vi "Tool Q LEIN stroke Stop Pressure Monitoring.vi"(1 "Retry on err (F)":bool, 11 "error in (no error)":errorcluster) -> (4 "LEIN custom reply Q":T1, 15 "error out":errorcluster)   [LabVIEW 2011]
uses:
  LEINmaster/Defenitions/LEIN custom reply Q.ctl
  LEINmaster/Defenitions/LEIN Reply Holder.ctl
  LEINmaster/Defenitions/LEIN CMD Cluster.ctl
  LEINmaster/Defenitions/LEIN CMD List.ctl
  LEINmaster/Defenitions/LEIN Structure variations.ctl
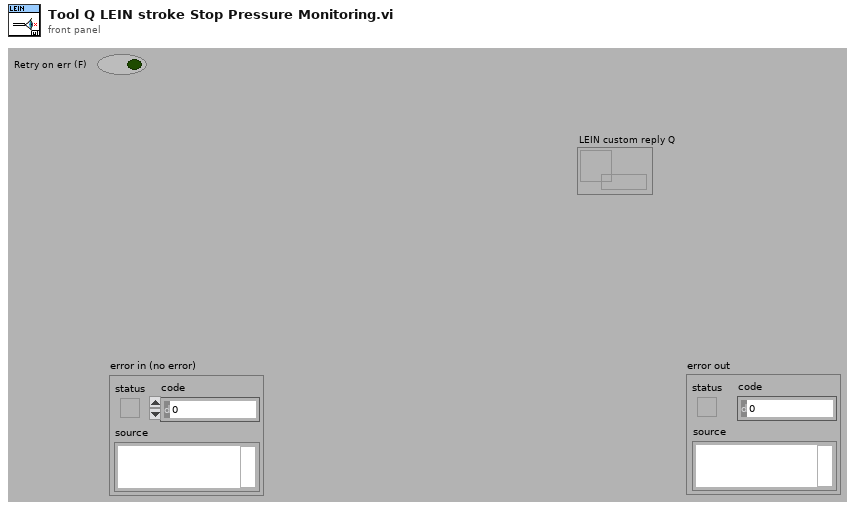
[diagram p1: front panel]
types:
  T1 = typedef "LEIN custom reply Q.ctl" = refnum<queue>
  T2 = typedef "LEIN Structure variations.ctl" = enum16{"LEIN08", "LEIN31", "LEIN63"}
  T3 = typedef "LEIN CMD Cluster.ctl" = cluster{"SID":u8, "ANF":bool, "CMD":T4, "DATA":u8[]}
  T4 = typedef "LEIN CMD List.ctl" = enum8{"ACTI", "TASK", "RES0", "STAT", "RES1", "RES2", "RES3", "USER"}
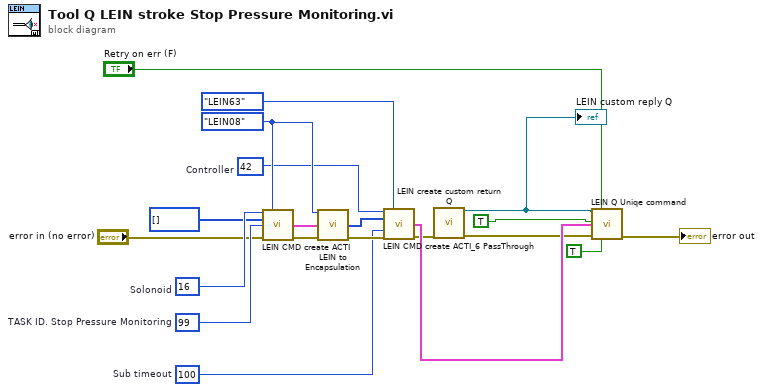
[diagram p0: block diagram]
diagram:
  w10 = u8 42  # Controller
  w11 = u8 16  # Solonoid
  w16 = u16 100  # Sub timeout
  w13 = u8 99  # TASK ID. Stop Pressure Monitoring
  w12 = LEIN_Structure_variations."LEIN08" ("LEIN Variation")
  n1 = call "LEIN CMD create ACTI.vi"("SID"=w11, "LEIN Variation"=w12, "Data"=u8[] [], "ACTI ID"=w13, "error in (no error)"="error in (no error)") -> ("CMD"=w14:T3, "error out"=w15:errorcluster)  [unwired: 9 in]
  n2 = call "LEIN to Encapsulation.vi"("LEIN Variation"=w12, "CMD"=w14, "error in (no error)"=w15) -> ("Data and header"=w17:u8[], "error out"=w18:errorcluster)  [unwired: 8 in, 3 out]
  n3 = call "LEIN CMD create ACTI_6 PassThrough.vi"("SID"=w10, "LEIN Variation"=LEIN_Structure_variations."LEIN63", "LEIN ecapsulated data (header and data)"=w17, "Sub Timeout (ms)"=w16, "error in (no error)"=w18) -> ("CMD"=w5:T3, "error out"=w4:errorcluster)  [unwired: 9 in]
  n4 = call "LEIN create custom return Q.vi"("error in (no error)"=w4) -> ("LEIN custom reply Q"=w2:T1, "error out"=w3:errorcluster)  [unwired: 13 in]
  "LEIN custom reply Q" <- w2
  n5 = call "LEIN Q Uniqe command.vi"("LEIN custom reply Q"=w2, "Retry on err (F)"="Retry on err (F)", "Custom Q(F)"=TRUE, "CMD"=w5, "error in"=w3, "priority(F)"=TRUE) -> ("error out"=→"error out":errorcluster)  [unwired: 9 in]
